vi "Search and connect.vi"(8 "error in":errorcluster) -> (0 "error out":errorcluster, 3 "VISA resource out":refnum<visa-resource-name>)   [LabVIEW 2021, in "F-70 driver.lvlib"]
doc: "Uses \"Find free COM ports\" and tries \"Initialize connection\" to find a compressor connected to a COM port.\nWhen no error occures, connection is established.\nIf error occures, connection is closed. Please check if the compressor is connected to a free COM port."
uses:
  F-70 driver.lvlib
  <vilib>/Utility/error.llb/Error Cluster From Error Code.vi
  <vilib>/ErrorRing/Error Ring.xnode
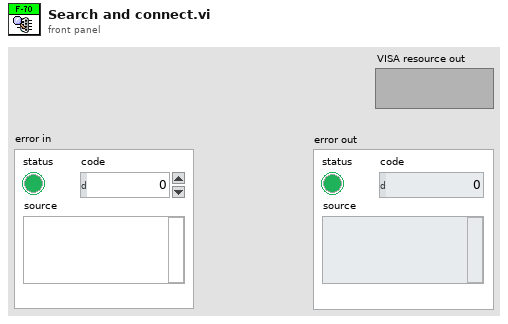
[diagram p1: front panel]
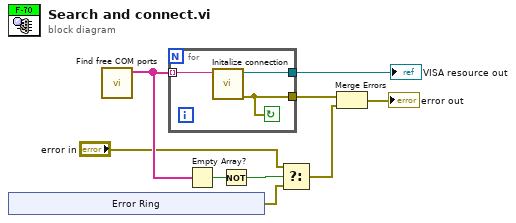
[diagram p0: block diagram]
diagram:
  n1 = xnode "Error Ring"() -> ("error out"=w4:errorcluster)
  n2 = call "Find free COM ports.vi"() -> ("Free COM ports"=w3:string[])  [unwired: 11 in]
  n3 = for {
    tunnel: w3 -> [w12] mode=indexing
    tunnel: [w11] -> w9
    tunnel: [w10] -> w8
    stop <- w10 continue-if-true
    n4 = call "Initalize connection.vi"("VISA resource in"=w12) -> ("error out"=w10:errorcluster, "VISA resource out"=w11:refnum<visa-resource-name>)  [unwired: 4 in, 1 out]
  }
  "VISA resource out" <- w9
  n5 = Empty Array?(array=w3) -> (empty?=w2:bool)
  n6 = Not(x=w2) -> (.not. x?=w7:bool)
  n7 = Select(t="error in", s=w7, f=w4) -> (s? t:f=w5:errorcluster)
  n8 = Merge Errors(w8, w5) -> (→"error out":errorcluster)
